vi "DumpImageSet (SubVI).vi"(6 "error in (no error)":errorcluster, 8 "Calibrated Image Array":T1[](array[typedef])) -> (0 "error out":errorcluster)   [LabVIEW 2016]
uses:
  <vilib>/vision/Image Controls.llb/IMAQ Image.ctl
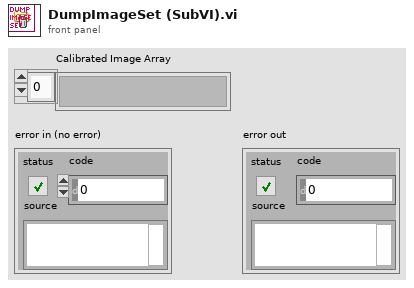
[diagram p1: front panel]
types:
  T1 = typedef "IMAQ Image.ctl" = refnum<image>
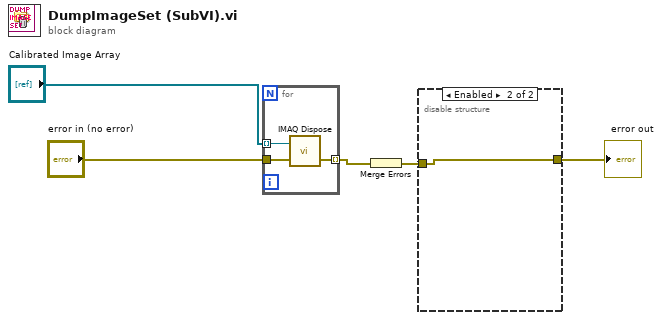
[diagram p0: block diagram]
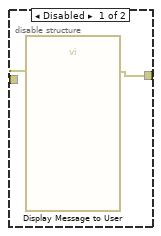
[diagram p2: hidden frame]
diagram:
  n1 = for {
    tunnel: "error in (no error)" -> [w8]
    tunnel: [w7] -> w2 mode=indexing
    tunnel: "Calibrated Image Array" -> [w6] mode=indexing
    n2 = call "IMAQ Dispose"("Image"=w6, "error in (no error)"=w8) -> ("error out"=w7:errorcluster)  [unwired: 4 in]
  }
  n3 = Merge Errors(w2) -> (w1:errorcluster)
  n4 = disable-structure shown="Enabled" {
    disable-tunnel: [w10 w11] -> w3
    disable-tunnel: w1 -> [w9 w11]
    frame Disabled {
      n5 = call "Display Message to User"("error in (no error)"=w9) -> ("error out"=w10:errorcluster)  [unwired: 9 in, 1 out]
    }
    frame Enabled {
    }
  }
  "error out" <- w3
